vi "Example Server.vi"() -> ()   [LabVIEW 2018, in "TCPServer.lvlib"]
uses:
  TCPServer.lvlib
  <vilib>/ErrorRing/Error Ring.xnode
  <vilib>/Utility/error.llb/Error Cluster From Error Code.vi
panel:
  in  "Stop":bool
  in  "TLM out":cluster{"VOLTAGE":dbl, "NAME[20]":string}={"VOLTAGE"=3.14, "NAME[20]"="Hello World"}
  out "CMD Packet":string
  out "CMD in":cluster{"CHANNEL":u8, "VALUE":dbl}
  out "Server Ports":u16[](array[numeric])
  out "Client IP:Ports":string[](array[string])
  out "Connected?":bool[](array[boolean])
  out "Internal Error":errorcluster
  in  "Send Tlm":bool
  out "Error":errorcluster
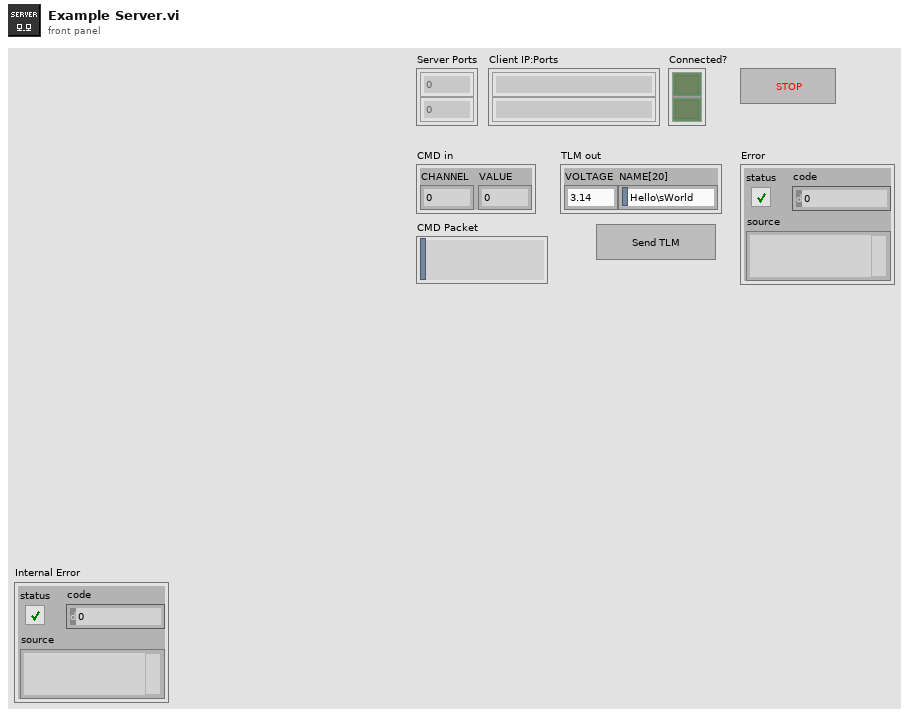
[diagram p1: front panel]
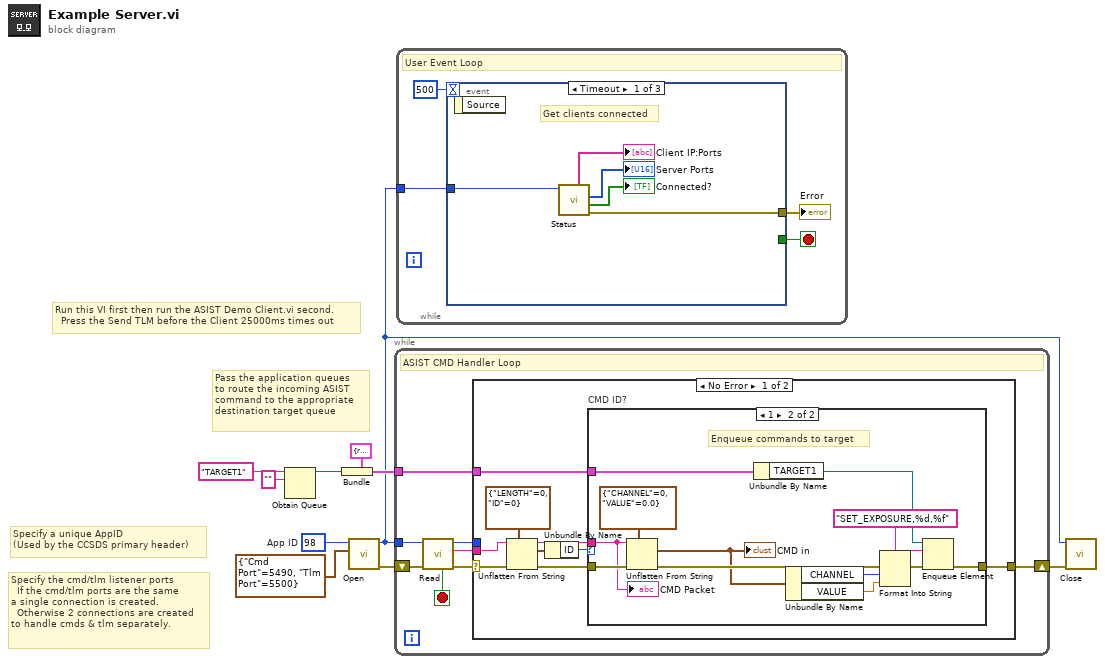
[diagram p0: block diagram]
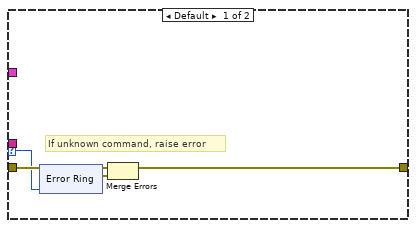
[diagram p2: hidden frame]
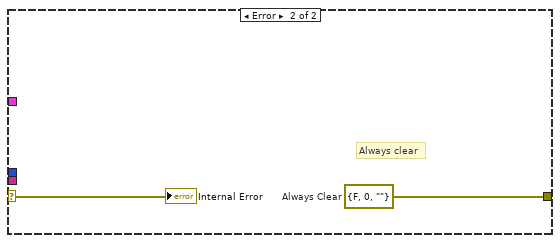
[diagram p3: hidden frame]
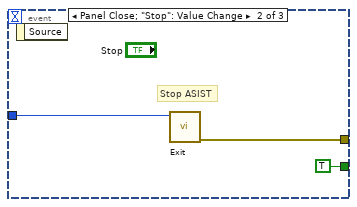
[diagram p4: hidden frame]
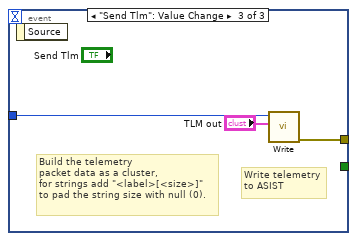
[diagram p5: hidden frame]
diagram:
  w10 = u16 98  # App ID
  # "Run this VI first then run the ASIST Demo Client.vi second.\n  Press the Send TLM before the Client 25000ms times out"
  # "Pass the application queues\nto route the incoming ASIST\ncommand to the appropriate\ndestination target queue"
  # "Specify a unique AppID\n(Used by the CCSDS primary header)"
  # "Specify the cmd/tlm listener ports\n  If the cmd/tlm ports are the same\na single connection is created.\n  Otherwise 2 connections are created\nto handle cmds & tlm separately."
  n1 = Obtain Queue(name (unnamed)="TARGET1", element data type="") -> (queue out=w4:refnum<queue>)  [unwired: 3 in, 2 out]
  n2 = Bundle(cluster=cluster{"TARGET1":refnum<queue>} {"TARGET1"=refnum} ("Queues"), "TARGET1"=w4) -> (w2:cluster{"TARGET1":refnum<queue>})
  n3 = call "Open.vi"("Ports (5123, 5123)"=cluster{"Cmd Port":u16, "Tlm Port":u16} {"Cmd Port"=5490, "Tlm Port"=5500} ("Ports"), "App ID in"=w10) -> ("error out"=w6:errorcluster, "App ID out"=w1:u16)  [unwired: 7 in, 1 out]
  n4 = while {
    tunnel: w1 -> [w12]
    tunnel: w2 -> [w17]
    shift-right: [w18] -> w5
    shift-left: w6 -> [w16]
    stop <- w11 stop-if-true
    # "ASIST CMD Handler Loop"
    n5 = call "Read.vi"("error in (no error)"=w16, "App ID in"=w12) -> ("error out"=w15:errorcluster, "Packet Data out"=w14:string, "App ID out"=w13:u16, "Exit?"=w11:bool)  [unwired: 5 in, 1 out]
    n6 = case shown="No Error" w15 {
      selector: w15 -> [w25 w52]
      tunnel: [w27 w53] -> w18
      tunnel: w17 -> [w26 _]
      tunnel: w14 -> [w23 _]
      tunnel: w13 -> [_ _]
      frame No Error {
        n7 = Unflatten From String(type=cluster{"LENGTH":i32, "ID":u16} {"LENGTH"=0, "ID"=0} ("Length"), binary string=w23, error in (no error)=w25) -> (rest of the binary string=w22:string, value=w20:cluster{"LENGTH":i32, "ID":u16}, error out=w24:errorcluster)  [unwired: 2 in]
        n8 = Unbundle By Name(w20) -> ("ID"=w19:u16)
        n9 = case "CMD ID?" shown="1" w19 {
          selector: w19 -> [w28 _]
          tunnel: w24 -> [w30 w48]
          tunnel: [w29 w47] -> w27
          tunnel: w26 -> [_ w46]
          tunnel: w22 -> [_ w39]
          frame Default {
            # "If unknown command, raise error"
            n10 = xnode "Error Ring"("parameter 0"=w28) -> ("error out"=w31:errorcluster)
            n11 = Merge Errors(w30, w31) -> (w29:errorcluster)
          }
          frame 1 {
            # "Enqueue commands to target"
            n12 = Unflatten From String(type=cluster{"CHANNEL":u8, "VALUE":dbl} {"CHANNEL"=0, "VALUE"=0.0}, binary string=w39, error in (no error)=w48) -> (value=w49:cluster{"CHANNEL":u8, "VALUE":dbl}, error out=w51:errorcluster)  [unwired: 2 in, 1 out]
            "CMD in" <- w49
            n13 = Unbundle By Name(w46) -> ("TARGET1"=w40:refnum<queue>)
            n14 = Unbundle By Name(w49) -> ("CHANNEL"=w42:u8, "VALUE"=w41:dbl)
            n15 = Format Into String(format string="SET_EXPOSURE,%d,%f", error in=w51, w42, w41) -> (resulting string=w43:string, error out=w45:errorcluster)  [unwired: 1 in]
            n16 = Enqueue Element(queue=w40, element=w43, error in (no error)=w45) -> (error out=w47:errorcluster)  [unwired: 1 in, 2 out]
            "CMD Packet" <- w39
          }
        }
      }
      frame Error {
        w53 = errorcluster {"status"=FALSE, "code"=0, "source"=""}  # Always Clear
        # "Always clear"
        "Internal Error" <- w52
      }
    }
  }
  n17 = while {
    tunnel: w1 -> [w54]
    stop <- w57 stop-if-true
    # "User Event Loop"
    n18 = event shown="[0] Timeout" {
      selector: _ -> [_ _ _]
      dyn-events: _ -> [_ _ _]
      timeout: 500 -> [_ _ _]
      tunnel: [_ TRUE ("Discard?") _] -> w57
      tunnel: [w62 w64 w68] -> w56
      tunnel: w54 -> [w61 w63 w66]
      event Timeout {
        # "Get clients connected"
        n19 = event-data() -> ()  [unwired: 1 in, 1 out]
        n20 = call "Status.vi"("App ID in"=w61) -> ("error out"=w62:errorcluster, "Connected?"=→"Connected?":bool[], "Server Ports"=→"Server Ports":u16[], "Client IP:Ports"=→"Client IP:Ports":string[])  [unwired: 4 in, 3 out]
      }
      event Panel Close; "Stop": Value Change {
        # "Stop ASIST"
        n21 = event-data() -> ()  [unwired: 1 in, 1 out]
        n22 = call "Exit.vi"("App ID in"=w63) -> ("error out"=w64:errorcluster)  [unwired: 9 in, 1 out]
      }
      event "Send Tlm": Value Change {
        # "Build the telemetry\npacket data as a cluster,\nfor strings add \"<label>[<size>]\"\nto pad the string size with null (0)."
        # "Write telemetry\nto ASIST"
        n23 = event-data() -> ()  [unwired: 1 in, 1 out]
        n24 = call "Write.vi"("Cluster"="TLM out", "App ID in"=w66) -> ("error out"=w68:errorcluster)  [unwired: 8 in, 1 out]
      }
    }
    "Error" <- w56
  }
  n25 = call "Close.vi"("error in (no error)"=w5, "App ID in"=w1) -> ()  [unwired: 9 in, 1 out]
